vi "LabVIEW Lib Paths.vi"() -> (1 "instr.lib":path, 2 "user.lib":path, 3 "vi.lib":path)   [LabVIEW 2016, in "Better Search.lvlib"]
uses:
  Better Search.lvlib
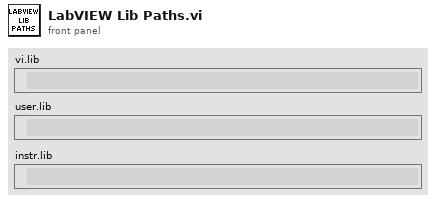
[diagram p1: front panel]
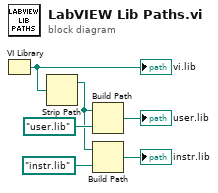
[diagram p0: block diagram]
diagram:
  n1 = VI Library() -> (path=w3:path)
  "vi.lib" <- w3
  n2 = Strip Path(path=w3) -> (stripped path=w4:path)  [unwired: 1 out]
  n3 = Build Path(base path=w4, name or relative path=path "user.lib") -> (appended path=→"user.lib":path)
  n4 = Build Path(base path=w4, name or relative path=path "instr.lib") -> (appended path=→"instr.lib":path)
